vi "MOD_STATE_FGV.vi"(7 "Write":bool, 8 "inMS3":T1 {"Angle"."SIN" format="%13.4f"; "Angle"."COS" format="%13.4f"; "Angle"."VALUE" format="%13.4f"}, 9 "inMS2":T1 {"Angle"."SIN" format="%13.4f"; "Angle"."COS" format="%13.4f"; "Angle"."VALUE" format="%13.4f"}, 10 "inMS1":T1 {"Angle"."SIN" format="%13.4f"; "Angle"."COS" format="%13.4f"; "Angle"."VALUE" format="%13.4f"}, 11 "inMS0":T1 {"Angle"."SIN" format="%13.4f"; "Angle"."COS" format="%13.4f"; "Angle"."VALUE" format="%13.4f"}) -> (0 "outMS3":T1 {"Angle"."SIN" format="%13.4f"; "Angle"."COS" format="%13.4f"; "Angle"."VALUE" format="%13.4f"}, 1 "outMS2":T1 {"Angle"."SIN" format="%13.4f"; "Angle"."COS" format="%13.4f"; "Angle"."VALUE" format="%13.4f"}, 2 "outMS1":T1 {"Angle"."SIN" format="%13.4f"; "Angle"."COS" format="%13.4f"; "Angle"."VALUE" format="%13.4f"}, 3 "outMS0":T1 {"Angle"."SIN" format="%13.4f"; "Angle"."COS" format="%13.4f"; "Angle"."VALUE" format="%13.4f"})   [LabVIEW 2019]
uses:
  <vilib>/Rock Robotics/WPI/ThirdParty/JAS_Junk/TrajLib/ROTATION2D.ctl
  <vilib>/Rock Robotics/WPI/ThirdParty/JAS_Junk/TrajLib/Trajectory_Library.lvlib
  <vilib>/Rock Robotics/WPI/ThirdParty/JAS_Junk/TrajLib/SWERVE_DRIVE_MODULE_STATE.ctl
panel:
  # "NON-REENTRANT\nON PURPOSE TO\nALLOW SAVING VALUES..."
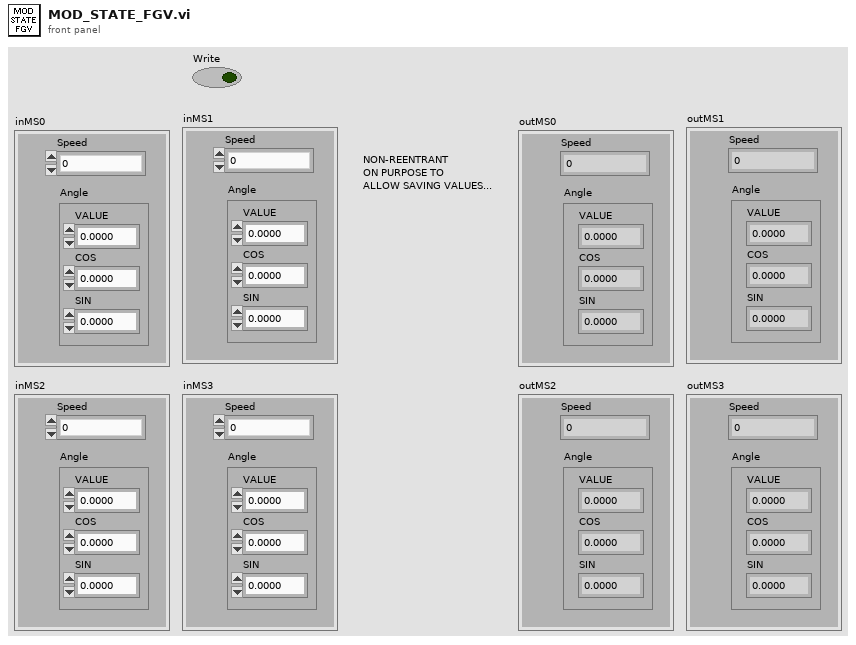
[diagram p1: front panel]
types:
  T1 = typedef "Trajectory_Library.lvlib/SWERVE_DRIVE_MODULE_STATE.ctl" = cluster{"Speed":dbl, "Angle":T2}
  T2 = typedef "Trajectory_Library.lvlib/ROTATION2D.ctl" = cluster{"VALUE":dbl, "COS":dbl, "SIN":dbl}
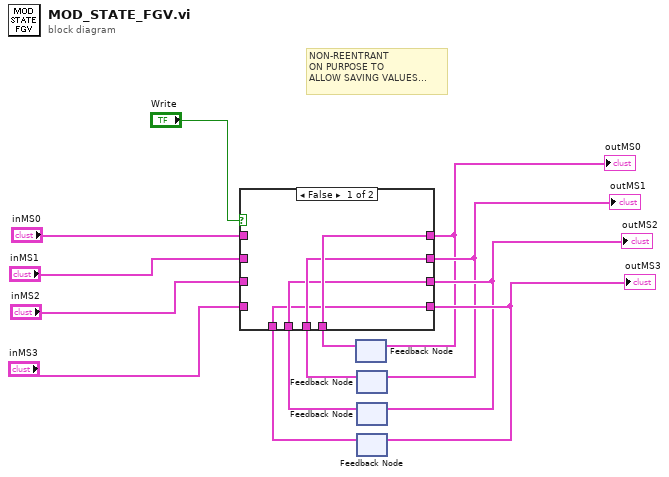
[diagram p0: block diagram]
diagram:
  # "NON-REENTRANT\nON PURPOSE TO\nALLOW SAVING VALUES..."
  n1 = feedback #1() -> (w10:T1)  [unwired: 1 in]
  n2 = feedback #2() -> (w11:T1)  [unwired: 1 in]
  n3 = feedback #3() -> (w12:T1)  [unwired: 1 in]
  n4 = feedback #4() -> (w13:T1)  [unwired: 1 in]
  n5 = case shown="False" "Write" {
    tunnel: "inMS0" -> [_ w21]
    tunnel: "inMS1" -> [_ w20]
    tunnel: "inMS2" -> [_ w19]
    tunnel: "inMS3" -> [_ w18]
    tunnel: [w17 w21] -> w6
    tunnel: [w16 w20] -> w7
    tunnel: [w15 w19] -> w8
    tunnel: [w14 w18] -> w9
    tunnel: w10 -> [w17 _]
    tunnel: w11 -> [w16 _]
    tunnel: w12 -> [w15 _]
    tunnel: w13 -> [w14 _]
    frame False {
    }
    frame True {
    }
  }
  "outMS3" <- w9
  "outMS2" <- w8
  "outMS1" <- w7
  "outMS0" <- w6
  n6 = feedback-in #1(w6) -> ()
  n7 = feedback-in #2(w7) -> ()
  n8 = feedback-in #3(w8) -> ()
  n9 = feedback-in #4(w9) -> ()
